vi "Cmd.ChangeProgram.vi"(6 "Timeout [ms] (1000)":i32=1000, 8 "error in":errorcluster, 9 "Program":u16 max=999, 10 "SDCard":u8=1 min=1 max=2, 11 "cID in":refnum<k5>) -> (0 "error out":errorcluster, 3 "cID out":refnum<k5>)   [LabVIEW 2016]
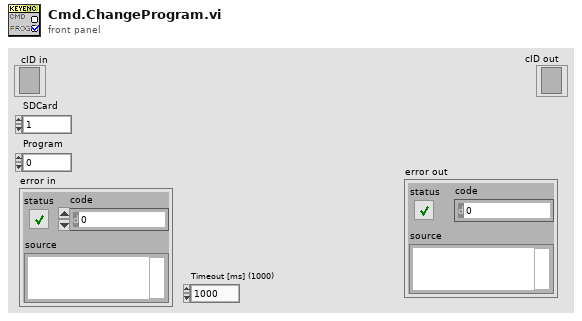
[diagram p1: front panel]
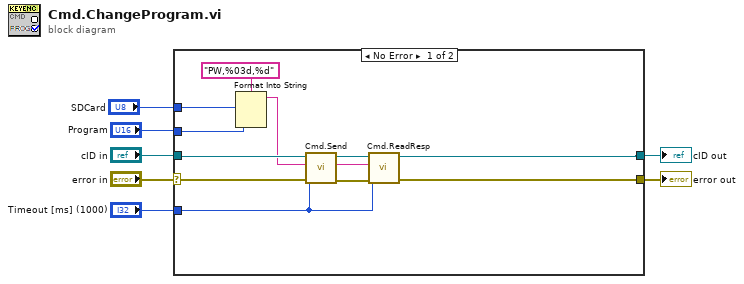
[diagram p0: block diagram]
diagram:
  n1 = case shown="No Error" "error in" {
    selector: "error in" -> [w17 w19]
    tunnel: "Timeout [ms] (1000)" -> [w12 _]
    tunnel: "cID in" -> [w18 w20]
    tunnel: [w11 w20] -> w4
    tunnel: [w10 w19] -> w3
    tunnel: "Program" -> [w9 _]
    tunnel: "SDCard" -> [w8 _]
    frame No Error {
      n2 = Format Into String(format string="PW,%03d,%d", w8, w9) -> (resulting string=w14:string)  [unwired: 2 in, 1 out]
      n3 = call "Cmd.Send.vi"("error in (no error)"=w17, "Timeout [ms] (1000)"=w12, "Command"=w14, "connection ID"=w18) -> ("error out"=w13:errorcluster, "connection ID out"=w15:refnum<k5>)  [unwired: 6 in]
      n4 = call "Cmd.ReadResp.vi"("error in (no error)"=w13, "Timeout [ms] (1000)"=w12, "Request"=w14, "connection ID"=w15) -> ("error out"=w10:errorcluster, "connection ID out"=w11:refnum<k5>)  [unwired: 5 in, 1 out]
    }
    frame Error {
    }
  }
  "cID out" <- w4
  "error out" <- w3
